vi "Key.vi"(4 "Comment (Create only)":string, 6 "Operation (Read or Create)":enum8{"Read or Create", "Read", "Write"}(ring), 7 "Section":string, 8 "error in (no error)":errorcluster, 9 "Value":string, 10 "Key":string, 11 "Ini Path in":path) -> (0 "error out":errorcluster, 1 "Found?":bool, 2 "Value out":string, 3 "Ini Path out":path)   [LabVIEW 2018, in "Config.lvlib"]
uses:
  Config.lvlib
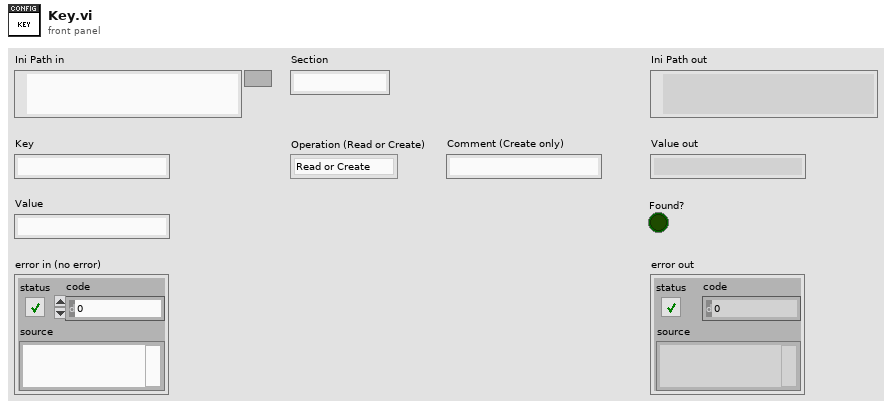
[diagram p1: front panel]
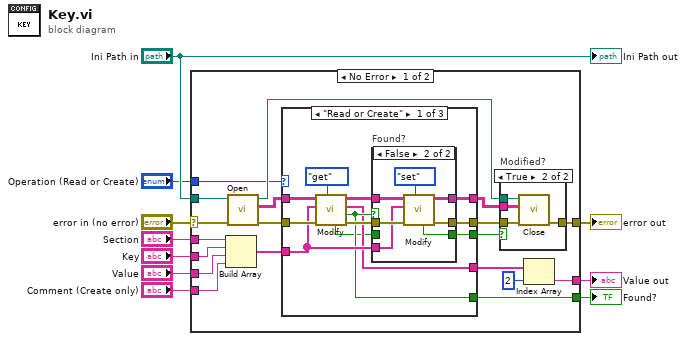
[diagram p0: block diagram]
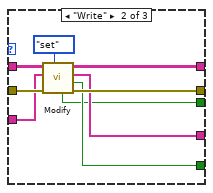
[diagram p3: hidden frame]
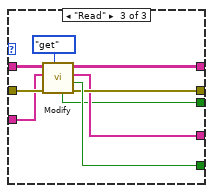
[diagram p4: hidden frame]
diagram:
  n1 = case shown="No Error" "error in (no error)" {
    selector: "error in (no error)" -> [w29 w76]
    tunnel: "Ini Path in" -> [w28 _]
    tunnel: "Section" -> [w25 _]
    tunnel: "Key" -> [w24 _]
    tunnel: "Value" -> [w23 w75]
    tunnel: "Comment (Create only)" -> [w22 _]
    tunnel: "Operation (Read or Create)" -> [w14 _]
    tunnel: [w12 w75] -> w3
    tunnel: [w15 _] -> w2
    tunnel: [w21 w76] -> w1
    frame No Error {
      n2 = Build Array(w25, w24, w23, w22) -> (w19:string[])
      n3 = call "Open.vi"("error in (no error)"=w29, "Ini Path in"=w28) -> ("error out"=w27:errorcluster, "skvc out"=w26:string[][], "Ini Path out"=w20:path)  [unwired: 6 in, 1 out]
      n4 = case shown="\"Read or Create\"" w14 {
        tunnel: w27 -> [w41 w60 w69]
        tunnel: w26 -> [w40 w59 w68]
        tunnel: w19 -> [w37 w58 w67]
        tunnel: [w36 w52 w61] -> w18
        tunnel: [w35 w57 w64] -> w17
        tunnel: [w34 w56 w63] -> w16
        tunnel: [w32 w54 w65] -> w15
        tunnel: [w31 w53 w62] -> w11
        frame "Read or Create" {
          n5 = call "Modify.vi"("Action (noop)"=enum8{"noop", "get", "set", "pop"}."get", "error in (no error)"=w41, "skvc input"=w37, "skvc in"=w40) -> ("error out"=w38:errorcluster, "Found?"=w32:bool, "skvc output"=w31:string[], "skvc out"=w39:string[][], "Modified?"=w30:bool)  [unwired: 3 in]
          n6 = case "Found?" shown="False" w32 {
            tunnel: w39 -> [w44 w51]
            tunnel: w38 -> [w43 w50]
            tunnel: w37 -> [_ w49]
            tunnel: [w42 w48] -> w36
            tunnel: [w43 w47] -> w35
            tunnel: [w44 w46] -> w34
            tunnel: w30 -> [w42 _]
            frame True {
            }
            frame False {
              n7 = call "Modify.vi"("Action (noop)"=enum8{"noop", "get", "set", "pop"}."set", "error in (no error)"=w50, "skvc input"=w49, "skvc in"=w51) -> ("error out"=w47:errorcluster, "skvc out"=w46:string[][], "Modified?"=w48:bool)  [unwired: 3 in, 2 out]
            }
          }
        }
        frame "Write" {
          n8 = call "Modify.vi"("Action (noop)"=enum8{"noop", "get", "set", "pop"}."set", "error in (no error)"=w60, "skvc input"=w58, "skvc in"=w59) -> ("error out"=w57:errorcluster, "Found?"=w54:bool, "skvc output"=w53:string[], "skvc out"=w56:string[][], "Modified?"=w52:bool)  [unwired: 3 in]
        }
        frame "Read" {
          n9 = call "Modify.vi"("Action (noop)"=enum8{"noop", "get", "set", "pop"}."get", "error in (no error)"=w69, "skvc input"=w67, "skvc in"=w68) -> ("error out"=w64:errorcluster, "Found?"=w65:bool, "skvc output"=w62:string[], "skvc out"=w63:string[][], "Modified?"=w61:bool)  [unwired: 3 in]
        }
      }
      n10 = case "Modified?" shown="True" w18 {
        tunnel: w17 -> [w70 w74]
        tunnel: [w70 w73] -> w21
        tunnel: w20 -> [_ w72]
        tunnel: w16 -> [_ w71]
        frame False {
        }
        frame True {
          n11 = call "Close.vi"("error in (no error)"=w74, "skvc in"=w71, "Ini Path in"=w72) -> ("error out"=w73:errorcluster)  [unwired: 7 in, 1 out]
        }
      }
      n12 = Index Array(array=w11, index=2) -> (element=w12:string)
    }
    frame Error {
    }
  }
  "error out" <- w1
  "Found?" <- w2
  "Value out" <- w3
  "Ini Path out" <- "Ini Path in"
